vi "FindLowest2Values.vi"(11 "Data Highway Out 2":T1={"New Image"=refnum, "Session Out"="", "LIDAR VISA Name"="", "Phidget Device Out"=0, "Lidar Data"=[], "polar attributes"={"maximum"=0.0, "minimum"=0.0, "clip to min"=FALSE, "log?(F)"=FALSE, "grid color"=6710886, "plot color"=65280, "fmt and prec"={"format"=enum."Decimal", "precision"=0}, "visible section"=8}, "Debug Message"="", "Servo Angles"={"Angle X"=0.0, "Angle Y"=0.0}, "ColorPlane"=refnum, "Threshold"=refnum, "PartFilt"=refnum, "Processed Image"=refnum, "Magnitude"=[], "Direction"=[]} {"polar attributes"."minimum" format="%0.2f"; "polar attributes"."maximum" format="%0.2f"}) -> (2 "Index of vals":i64[](array[numeric]), 3 "Data Highway Out 3":T1={"New Image"=refnum, "Session Out"="", "LIDAR VISA Name"="", "Phidget Device Out"=0, "Lidar Data"=[], "polar attributes"={"maximum"=0.0, "minimum"=0.0, "clip to min"=FALSE, "log?(F)"=FALSE, "grid color"=6710886, "plot color"=65280, "fmt and prec"={"format"=enum."Decimal", "precision"=0}, "visible section"=8}, "Debug Message"="", "Servo Angles"={"Angle X"=0.0, "Angle Y"=0.0}, "ColorPlane"=refnum, "Threshold"=refnum, "PartFilt"=refnum, "Processed Image"=refnum, "Magnitude"=[], "Direction"=[]} {"polar attributes"."minimum" format="%0.2f"; "polar attributes"."maximum" format="%0.2f"})   [LabVIEW 2014]
uses:
  controls/Data.ctl
  <vilib>/vision/Image Controls.llb/IMAQ Image.ctl
  <vilib>/userdefined/High Color/IMAQdx.ctl
panel:
  out "Pre-Transform":dbl[](graph)
  out "Post-Transform":dbl[](graph)
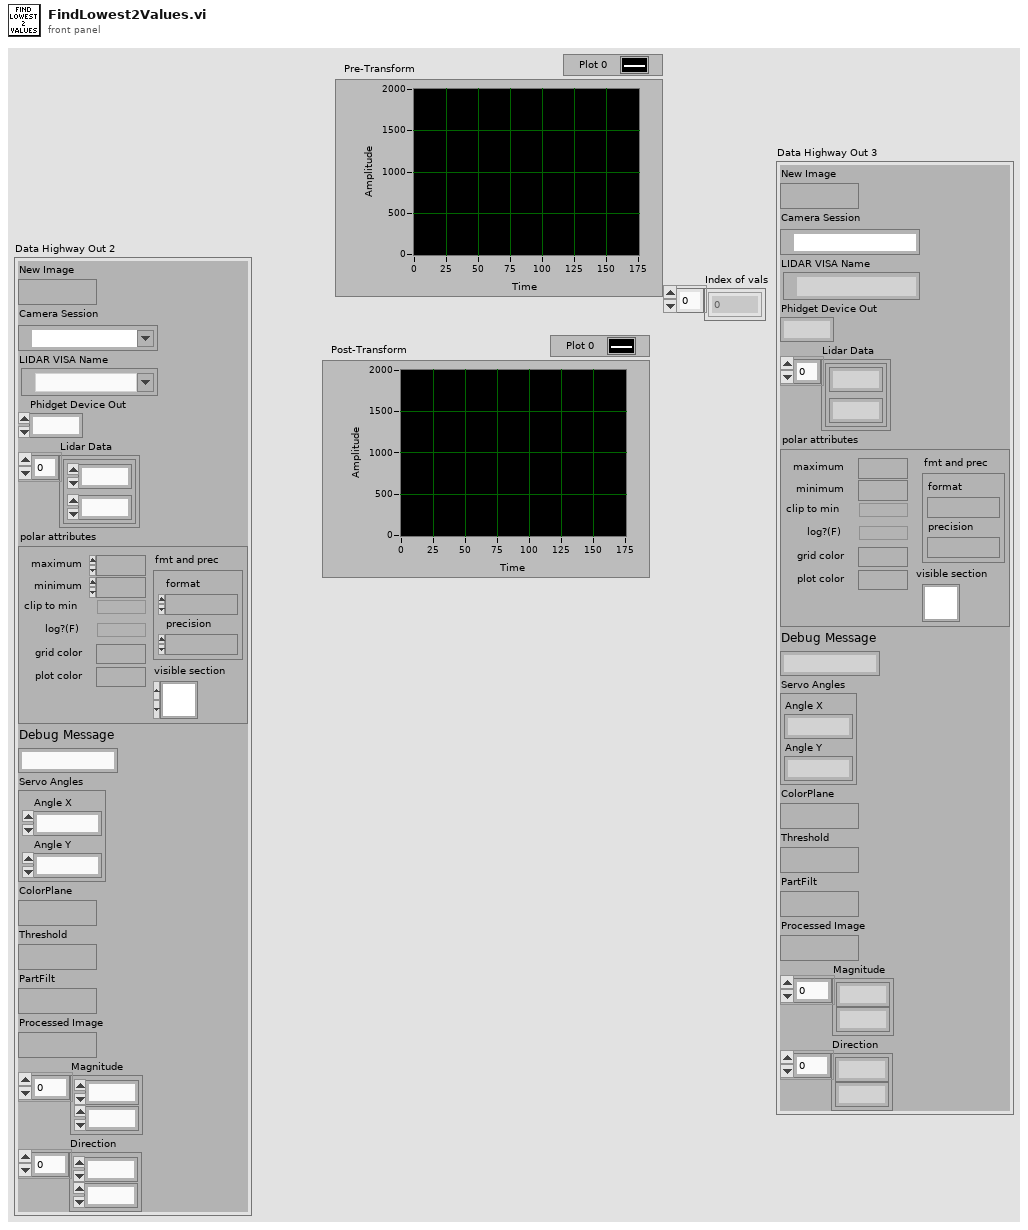
[diagram p1: front panel]
types:
  T1 = typedef "Data.ctl" = cluster{"New Image":T2, "Session Out":T3, "LIDAR VISA Name":refnum<visa-resource-name>, "Phidget Device Out":i32, "Lidar Data":cluster{dbl, dbl}[], "polar attributes":cluster{"maximum":dbl, "minimum":dbl, "clip to min":bool, "log?(F)":bool, "grid color":u32, "plot color":u32, "fmt and prec":cluster{"format":enum8{"Decimal", "Scientific", "Engineering", "Binary", "Octal", "Hex"}, "precision":u8}, "visible section":u16}, "Debug Message":string, "Servo Angles":cluster{"Angle X":dbl, "Angle Y":dbl}, "ColorPlane":T2, "Threshold":T2, "PartFilt":T2, "Processed Image":T2, "Magnitude":dbl[], "Direction":dbl[]}
  T2 = typedef "IMAQ Image.ctl" = refnum<image>
  T3 = typedef "IMAQdx.ctl" = refnum<k21>
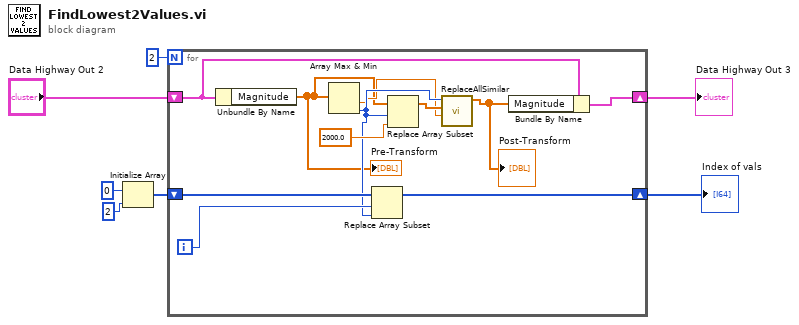
[diagram p0: block diagram]
diagram:
  n1 = Initialize Array(i64 0 ("element"), 2 ("dimension size")) -> (w3:i64[])
  n2 = for {
    N: 2 -> [_]
    shift-right: [w16] -> w1
    shift-left: w3 -> [w17]
    shift-right: [w14] -> w2
    shift-left: "Data Highway Out 2" -> [w15]
    i -> [w13]
    n3 = Unbundle By Name(w15) -> ("Magnitude"=w8:dbl[])
    "Pre-Transform" <- w8
    n4 = Array Max & Min(array=w8) -> (min value=w10:dbl, min index (indices)=w11:i32)  [unwired: 2 out]
    n5 = Replace Array Subset(array=w17, new element=w11, index=w13) -> (w16:i64[])
    n6 = Replace Array Subset(array=w8, new element=2000.0 ("new element/subarray"), index=w11) -> (w12:dbl[])
    n7 = call "ReplaceAllSimilar.vi"("min value"=w10, "Magnitude array"=w12, "min index(es)"=w11) -> ("Magnitude array 2"=w9:dbl[])  [unwired: 8 in]
    "Post-Transform" <- w9
    n8 = Bundle By Name(cluster=w15, "Magnitude"=w9) -> (w14:T1)
  }
  "Data Highway Out 3" <- w2
  "Index of vals" <- w1
